vi "SendCommand.vi"(6 "error in":errorcluster, 8 "Parameter":sgl, 9 "Command":u8, 10 "Address":u8, 11 "VISA resource name":refnum<visa-resource-name>) -> (0 "error out":errorcluster, 2 "return count":u32, 3 "VISA resource name out":refnum<visa-resource-name>)   [LabVIEW 2020, in "driver_flodx_ph_probe.lvlib"]
uses:
  <instrlib>/RxnRover/FloDx Ph Probe Driver/driver_flodx_ph_probe.lvlib
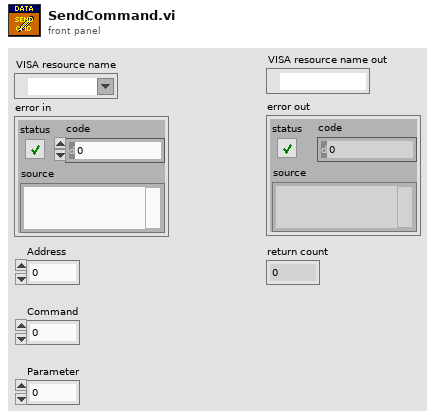
[diagram p1: front panel]
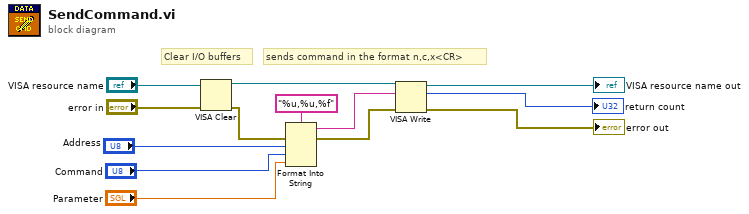
[diagram p0: block diagram]
diagram:
  # "Clear I/O buffers"
  # "sends command in the format n,c,x<CR>"
  n1 = VISA Clear(VISA resource name="VISA resource name", error in (no error)="error in") -> (VISA resource name out=w4:refnum<visa-resource-name>, error out=w2:errorcluster)
  n2 = Format Into String(format string="%u,%u,%f", error in=w2, "Address", "Command", "Parameter") -> (resulting string=w1:string, error out=w12:errorcluster)  [unwired: 1 in]
  n3 = VISA Write(VISA resource name=w4, write buffer=w1, error in (no error)=w12) -> (VISA resource name out=→"VISA resource name out":refnum<visa-resource-name>, return count=→"return count":u32, error out=→"error out":errorcluster)
